vi "Fire Update Event.vi"(6 "Sync Response":refnum<notifier>, 8 "error in (no error)":errorcluster, 10 "Synced":bool, 11 "2DArrayManager in":refnum<class "2DArrayManager.lvclass">) -> (0 "error out":errorcluster, 3 "2DArrayManager out":refnum<class "2DArrayManager.lvclass">)   [LabVIEW 2020, in "OOPanel.lvlib" / "2DArrayManager.lvclass"]
uses:
  2DArrayManager.lvclass
  Update Data.ctl
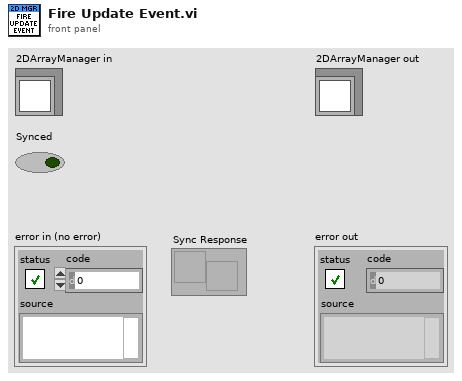
[diagram p1: front panel]
types:
  T1 = typedef "OOPanel.lvlib/2DArrayManager.lvclass/Update Data.ctl" = cluster{"Synced":bool, "Sync Response":refnum<notifier>}
  T2 = typedef "OOPanel.lvlib/2DArrayManager.lvclass/Event Reg Ref.ctl" = cluster{"Last Update Ticks ms":u32, "Event Reg":refnum<event-registration>}
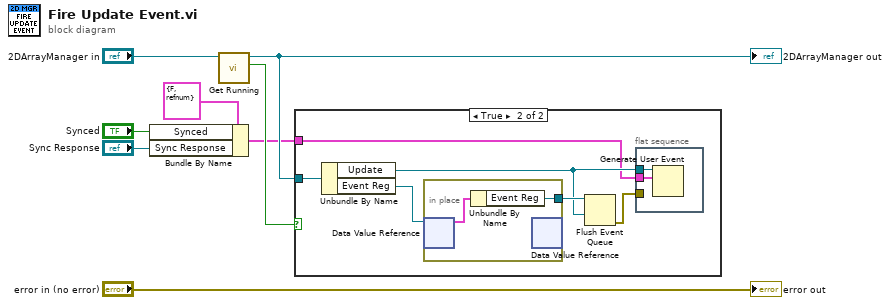
[diagram p0: block diagram]
diagram:
  n1 = Bundle By Name(cluster=T1 {"Synced"=FALSE, "Sync Response"=refnum} ("Update Data"), "Synced"="Synced", "Sync Response"="Sync Response") -> (w4:T1)
  n2 = call "Get Running.vi"("2DArrayManager in"="2DArrayManager in") -> ("Running"=w8:bool, "2DArrayManager out"=w6:refnum<class "2DArrayManager.lvclass">)  [unwired: 8 in, 1 out]
  "2DArrayManager out" <- w6
  n3 = case shown="True" w8 {
    tunnel: w6 -> [_ w14]
    tunnel: w4 -> [_ w9]
    frame False {
    }
    frame True {
      n4 = Unbundle By Name(w14) -> ("Update"=w11:refnum<user-event>, "Event Reg"=w13:refnum<data-value>)
      n5 = in-place {
        in-place-border: [w17] -> w12
        n6 = in-place-dvr #1(w13) -> (w18:T2)  [unwired: 1 out]
        n7 = Unbundle By Name(w18) -> ("Event Reg"=w17:refnum<event-registration>)
        n8 = in-place-dvr #1() -> ()  [unwired: 1 in, 2 out]
      }
      n9 = Flush Event Queue(0:w12, 2:w11) -> (11:w10:errorcluster)  [unwired: 4 in, 2 out]
      n10 = flat-sequence {
        tunnel: w11 -> [w16]
        tunnel: w10 -> [_]
        tunnel: w9 -> [w15]
        frame #0 {
          n11 = Generate User Event(user event=w16, event data cluster=w15) -> ()  [unwired: 2 in, 2 out]
        }
      }
    }
  }
  "error out" <- "error in (no error)"
